vi "SIM_FrameProperties.vi"() -> (0 "data":dbl[][](array[numeric]), 3 "Frame Properties":T1)   [LabVIEW 2017]
uses:
  GlobalClicksHeight.vi
  <vilib>/Utility/file.llb/Read Delimited Spreadsheet (DBL).vi
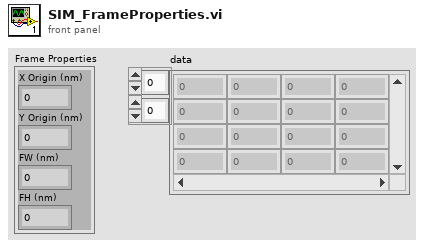
[diagram p1: front panel]
types:
  T1 = cluster{"X Origin (nm)":dbl, "Y Origin (nm)":dbl, "FW (nm)":dbl, "FH (nm)":dbl}
  T2 = cluster{"array[0]":i32, "array[1]":i32, "array[2]":i32, "array[3]":i32, "array[4]":i32, "array[5]":i32, "array[6]":i32, "array[7]":i32, "array[8]":i32}
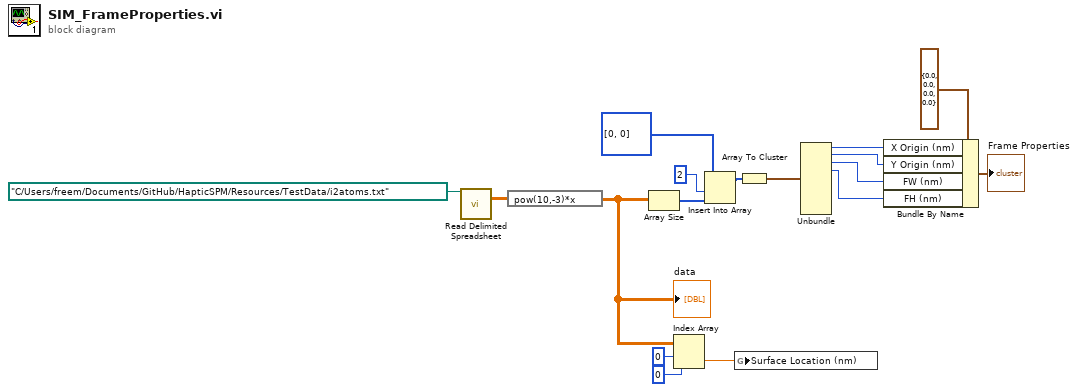
[diagram p0: block diagram]
diagram:
  n1 = call-poly <vilib>:"Read Delimited Spreadsheet.vi"("file path (dialog if empty)"=path "C:/Users/freem/Documents/GitHub/HapticSPM/Resources/TestData/i2atoms.txt") -> ("all rows"=w2:dbl[][])  [unwired: 9 in, 5 out]
  n2 = expression code="pow(10,-3)*x"(w2) -> (w1:dbl[][])
  "data" <- w1
  n3 = Array Size(array=w1) -> (size(s)=w7:i32[])
  n4 = Index Array(array=w1, index (row)=0, index (col)=0 ("disabled index (col)")) -> (element=w4:dbl)
  n5 = Insert Into Array(array=i32[] [0, 0], index=2, new element=w7) -> (w15:i32[])
  n6 = global write "GlobalClicksHeight.vi" "Surface Location (nm)"(w4) -> ()
  n7 = Array To Cluster(array=w15) -> (cluster=w14:T2)
  n8 = Unbundle(w14) -> ("array[0]"=w12:i32, "array[1]"=w11:i32, "array[2]"=w10:i32, "array[3]"=w9:i32)  [unwired: 5 out]
  n9 = Bundle By Name(cluster=T1 {"X Origin (nm)"=0.0, "Y Origin (nm)"=0.0, "FW (nm)"=0.0, "FH (nm)"=0.0} ("Frame Properties (Remapped)"), "X Origin (nm)"=w12, "Y Origin (nm)"=w11, "FW (nm)"=w10, "FH (nm)"=w9) -> (→"Frame Properties":T1)
